vi "Calibrate.vi"(8 "error in (no error)":errorcluster, 11 "Message Queue":refnum<queue>) -> (0 "error out":errorcluster)   [LabVIEW 2020, in "plugin_flodx_ph_probe.lvlib" / "plugin.lvlib"]
doc: "UI which prompts the user to calibrate the device, in two-point and three-point modes."
uses:
  plugin.lvlib
  <userlib>/RxnRover/PluginCore/src/support/Message Queue/Message Cluster.ctl
  <userlib>/RxnRover/PluginCore/src/support/Message Queue/Message Queue.lvlib
panel:
  in  "SHUTDOWN":bool
  in  "Compensation Temperature":sgl=25.0
  in  "Calibrate Button":bool
  in  "Calibration Method":enum32{"TWO-POINT", "THREE-POINT"}(radio)
  in  "Alkaline Buffer pH":sgl=9.8 min=0 format="%#_4g"
  in  "Neutral Buffer pH":sgl=7.01 min=0 format="%#_4g"
  in  "Acidic Buffer pH":sgl=4.1 format="%#_4g"
  in  "Cancel Button":bool
  # "Calibrate Device"
  # "To calibrate your device please input the pH of your buffer solutions used during calibration then choose one of the following options. (If you are only using two out of the three buffer solutions to calibrate leave the unused buffer pH value blank or enter 0)"
  # "Compensation Temperature (C)"
  # "(Calibration Standard 4.10)"
  # "Acidic Buffer(Low)"
  # "(Calibration Standard 7.01)"
  # "Neutral Buffer(Mid)"
  # "(Calibration Standard 9.80)"
  # "Alkaline Buffer(High)"
  # "Calibration Method"
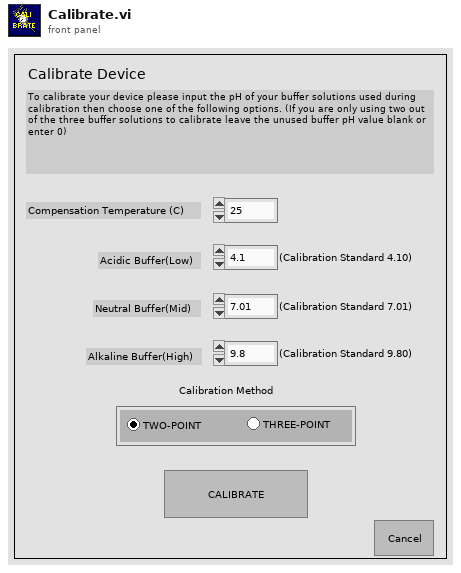
[diagram p1: front panel]
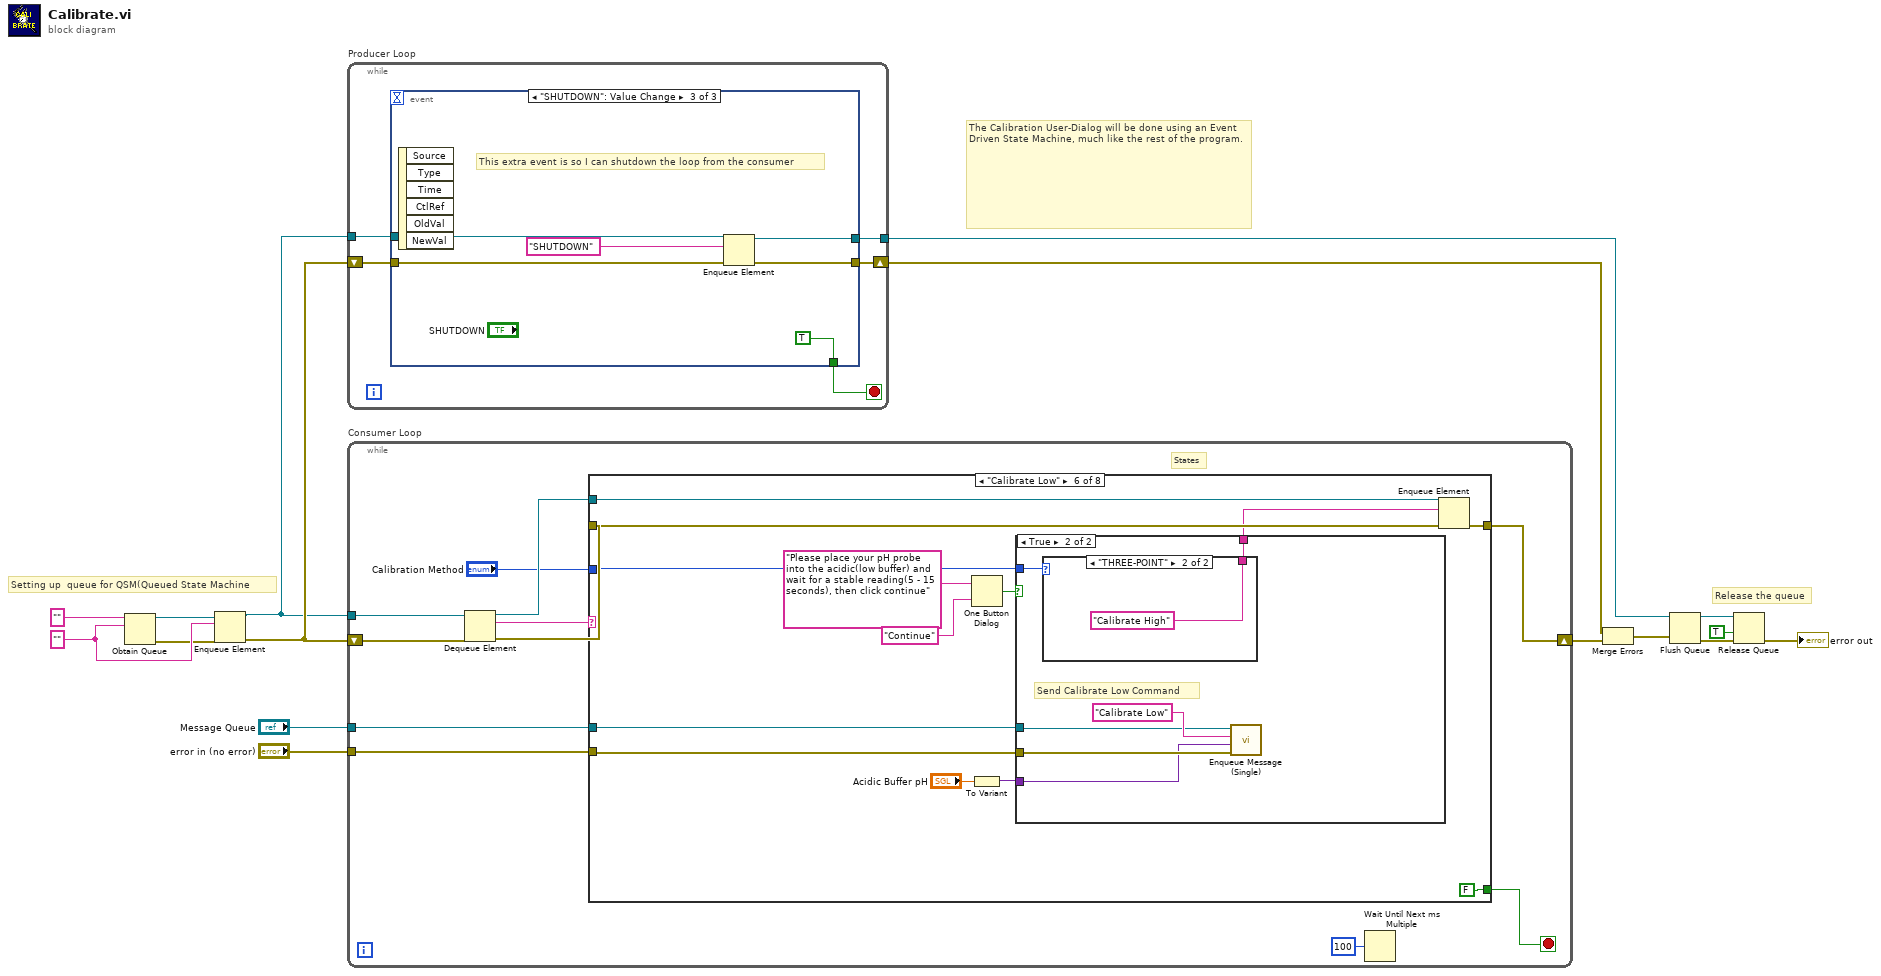
[diagram p0: block diagram]
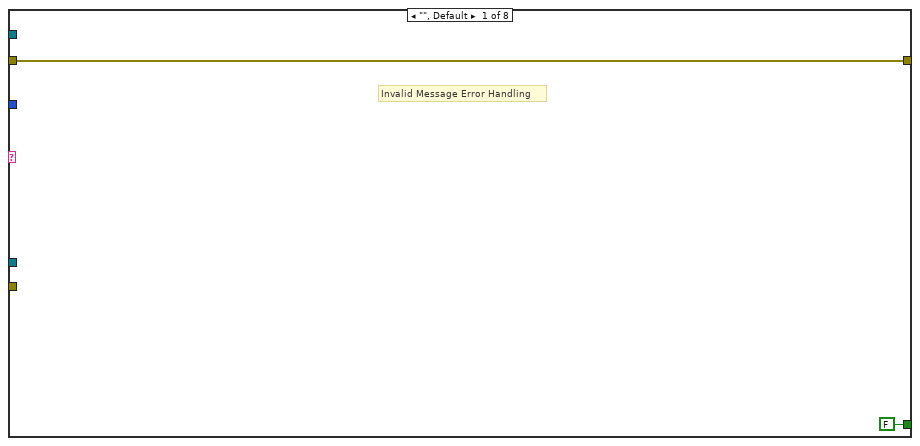
[diagram p2: hidden frame]
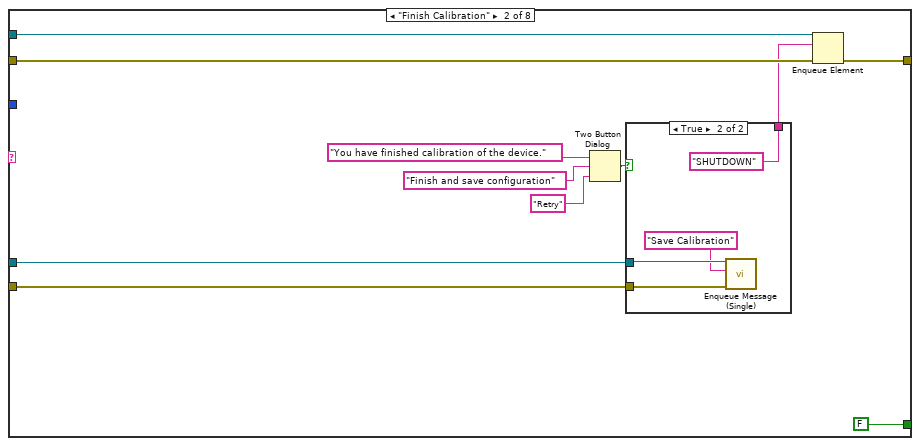
[diagram p3: hidden frame]
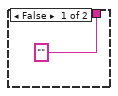
[diagram p4: hidden frame]
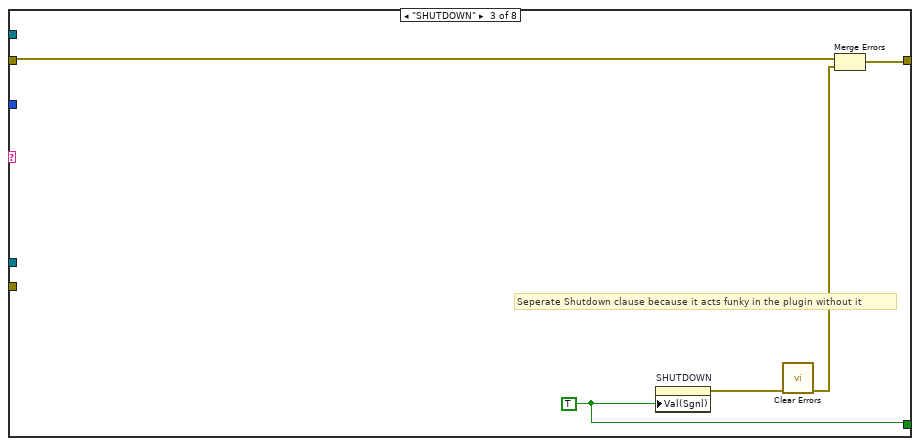
[diagram p5: hidden frame]
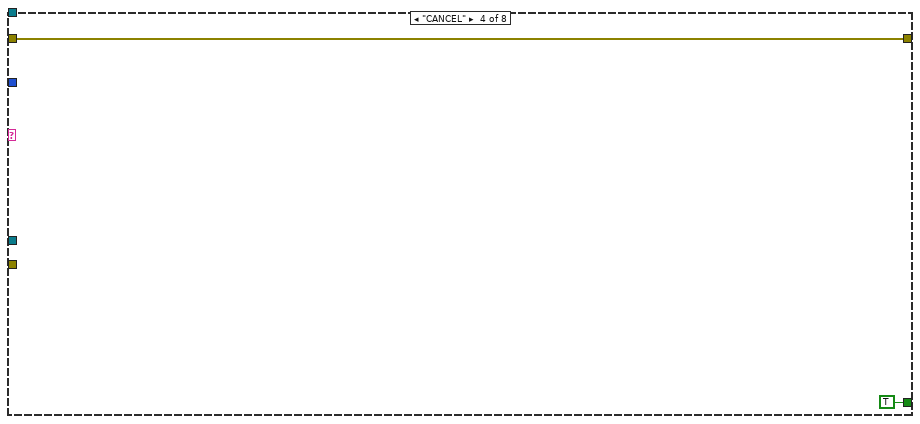
[diagram p6: hidden frame]
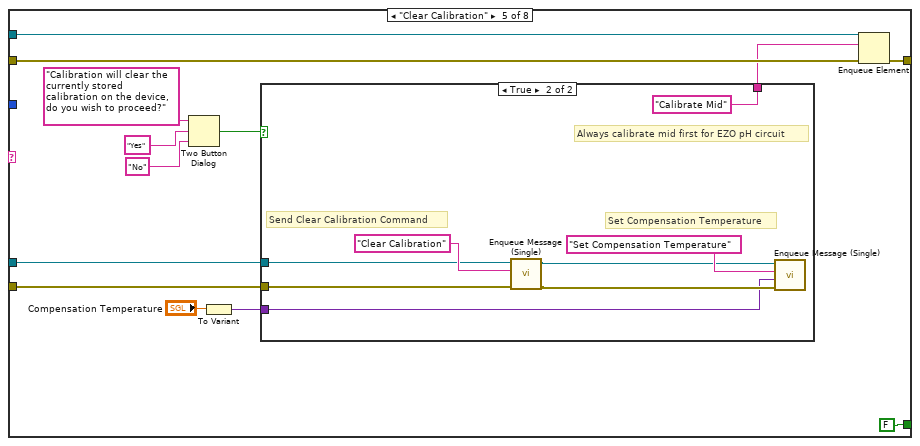
[diagram p7: hidden frame]
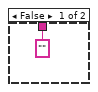
[diagram p8: hidden frame]
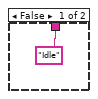
[diagram p9: hidden frame]
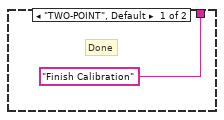
[diagram p10: hidden frame]
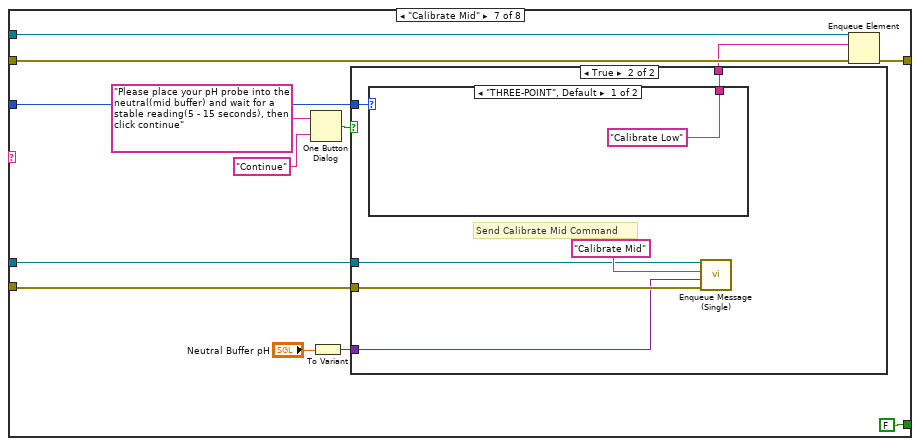
[diagram p11: hidden frame]
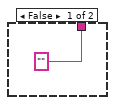
[diagram p12: hidden frame]
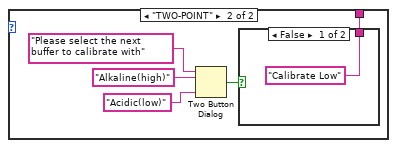
[diagram p13: hidden frame]
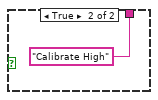
[diagram p14: hidden frame]
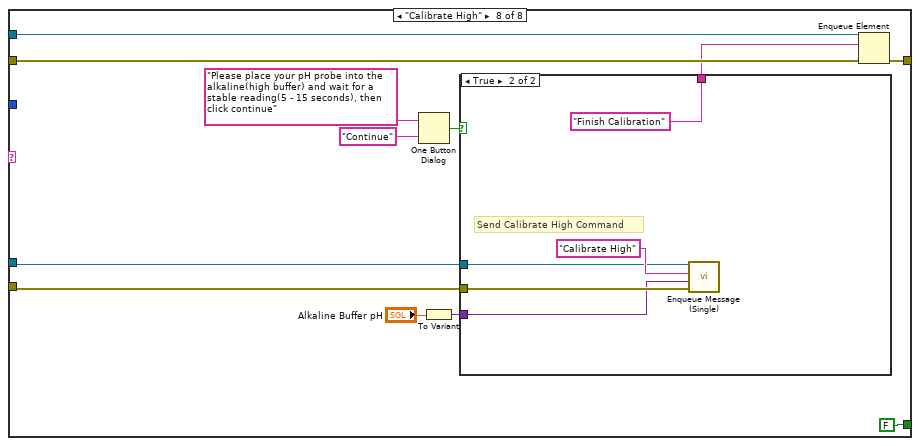
[diagram p15: hidden frame]
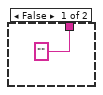
[diagram p16: hidden frame]
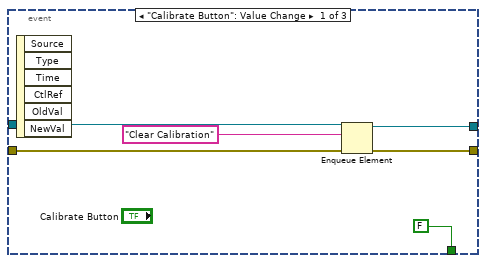
[diagram p17: hidden frame]
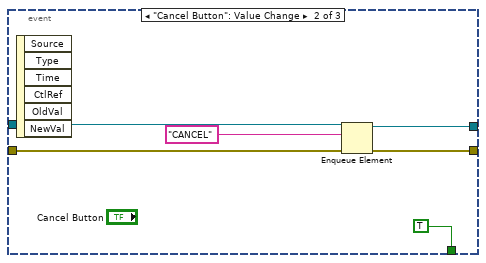
[diagram p18: hidden frame]
diagram:
  w15 = ""
  # "The Calibration User-Dialog will be done using an Event Driven State Machine, much like the rest of the program."
  # "Release the queue"
  # "Setting up  queue for QSM(Queued State Machine"
  n1 = Obtain Queue(name (unnamed)="", element data type=w15) -> (queue out=w14:refnum<queue>, error out=w13:errorcluster)  [unwired: 3 in, 1 out]
  n2 = Enqueue Element(queue=w14, element=w15, error in (no error)=w13) -> (queue out=w1:refnum<queue>, error out=w12:errorcluster)  [unwired: 1 in, 1 out]
  n3 = while "Producer Loop" {
    tunnel: w1 -> [w20]
    shift-right: [w18] -> w8
    shift-left: w12 -> [w21]
    tunnel: [w17] -> w6
    stop <- w19 stop-if-true
    n4 = event shown="[2] \"SHUTDOWN\": Value Change" {
      selector: _ -> [_ _ _]
      dyn-events: _ -> [_ _ _]
      timeout: _ -> [_ _ _]
      tunnel: w21 -> [w27 w33 w39]
      tunnel: w20 -> [w26 w32 w38]
      tunnel: [w25 w31 w37] -> w17
      tunnel: [FALSE TRUE TRUE] -> w19
      tunnel: [w22 w28 w34] -> w18
      event "Calibrate Button": Value Change {
        n5 = event-data() -> ()  [unwired: 1 in, 6 out]
        n6 = Enqueue Element(queue=w26, element="Clear Calibration", error in (no error)=w27) -> (queue out=w25:refnum<queue>, error out=w22:errorcluster)  [unwired: 1 in, 1 out]
      }
      event "Cancel Button": Value Change {
        n7 = event-data() -> ()  [unwired: 1 in, 6 out]
        n8 = Enqueue Element(queue=w32, element="CANCEL", error in (no error)=w33) -> (queue out=w31:refnum<queue>, error out=w28:errorcluster)  [unwired: 1 in, 1 out]
      }
      event "SHUTDOWN": Value Change {
        # "This extra event is so I can shutdown the loop from the consumer"
        n9 = event-data() -> ()  [unwired: 1 in, 6 out]
        n10 = Enqueue Element(queue=w38, element="SHUTDOWN", error in (no error)=w39) -> (queue out=w37:refnum<queue>, error out=w34:errorcluster)  [unwired: 1 in, 1 out]
      }
    }
  }
  n11 = while "Consumer Loop" {
    tunnel: w1 -> [w50]
    tunnel: "Message Queue" -> [w45]
    tunnel: "error in (no error)" -> [w44]
    shift-right: [w41] -> w9
    shift-left: w12 -> [w40]
    stop <- w46 stop-if-true
    # "States"
    n12 = Dequeue Element(queue=w50, error in (no error)=w40) -> (queue out=w48:refnum<queue>, element=w49:string, error out=w47:errorcluster)  [unwired: 1 in, 1 out]
    n13 = case shown="\"Calibrate Low\"" w49 {
      tunnel: w48 -> [_ w58 _ _ w88 w108 w130 w157]
      tunnel: w47 -> [w51 w59 w72 w74 w87 w107 w129 w156]
      tunnel: [FALSE ("T button?") FALSE ("T button?") w69 TRUE ("T button?") FALSE FALSE FALSE FALSE] -> w46
      tunnel: w45 -> [_ w60 _ _ w83 w110 w132 w159]
      tunnel: w44 -> [_ w61 _ _ w84 w109 w131 w158]
      tunnel: "Calibration Method" -> [_ _ _ _ _ w102 w124 _]
      tunnel: [w51 w56 w73 w74 w82 w100 w122 w150] -> w41
      frame "", Default {
        # "Invalid Message Error Handling"
      }
      frame "Finish Calibration" {
        n14 = Two Button Dialog(message="You have finished calibration of the device.", 1:"Retry" ("F button name (\"Cancel\")"), 2:"Finish and save configuration" ("T button name (\"OK\")")) -> (T button?=w55:bool)
        n15 = case shown="True" w55 {
          tunnel: w61 -> [_ w68]
          tunnel: w60 -> [_ w67]
          tunnel: ["" ("element") "SHUTDOWN" ("element")] -> w57
          frame False {
          }
          frame True {
            n16 = call <userlib>:"Enqueue Message (Single).vi"("error in (no error)"=w68, "Message"="Save Calibration", "Message Queue"=w67) -> ()  [unwired: 7 in, 2 out]
          }
        }
        n17 = Enqueue Element(queue=w58, element=w57, error in (no error)=w59) -> (error out=w56:errorcluster)  [unwired: 1 in, 2 out]
      }
      frame "SHUTDOWN" {
        w69 = TRUE
        # "Seperate Shutdown clause because it acts funky in the plugin without it"
        n18 = property on="SHUTDOWN" class="Bool (strict)"("Val(Sgnl)"=w69) -> (error out=w70:errorcluster)  [unwired: 2 in, 1 out]
        n19 = call <vilib>:"Clear Errors.vi"("error in (no error)"=w70) -> ("error out"=w71:errorcluster)  [unwired: 5 in, 1 out]
        n20 = Merge Errors(w72, w71) -> (w73:errorcluster)
      }
      frame "CANCEL" {
      }
      frame "Clear Calibration" {
        n21 = Two Button Dialog(message="Calibration will clear the currently stored calibration on the device, do you wish to proceed?", 1:"No" ("F button name (\"Cancel\")"), 2:"Yes" ("T button name (\"OK\")")) -> (T button?=w79:bool)
        n22 = To Variant(anything="Compensation Temperature") -> (Variant=w80:variant)
        n23 = case shown="True" w79 {
          tunnel: ["" ("element") "Calibrate Mid" ("element")] -> w86
          tunnel: w84 -> [_ w94]
          tunnel: w83 -> [_ w91]
          tunnel: w80 -> [_ w90]
          frame False {
          }
          frame True {
            # "Send Clear Calibration Command"
            # "Always calibrate mid first for EZO pH circuit"
            # "Set Compensation Temperature"
            n24 = call <userlib>:"Enqueue Message (Single).vi"("error in (no error)"=w94, "Message"="Clear Calibration", "Message Queue"=w91) -> ("error out"=w93:errorcluster, "dup Message Queue"=w92:refnum<queue>)  [unwired: 7 in]
            n25 = call <userlib>:"Enqueue Message (Single).vi"("error in (no error)"=w93, "Message Data"=w90, "Message"="Set Compensation Temperature", "Message Queue"=w92) -> ()  [unwired: 6 in, 2 out]
          }
        }
        n26 = Enqueue Element(queue=w88, element=w86, error in (no error)=w87) -> (error out=w82:errorcluster)  [unwired: 1 in, 2 out]
      }
      frame "Calibrate Low" {
        n27 = One Button Dialog(message="Please place your pH probe into the acidic(low buffer) and wait for a stable reading(5 - 15 seconds), then click continue", button name ("OK")="Continue") -> (true=w103:bool)
        n28 = To Variant(anything="Acidic Buffer pH") -> (Variant=w98:variant)
        n29 = case shown="True" w103 {
          tunnel: w110 -> [_ w116]
          tunnel: w109 -> [_ w115]
          tunnel: ["Idle" ("element") w114] -> w106
          tunnel: w102 -> [_ w113]
          tunnel: w98 -> [_ w112]
          frame False {
          }
          frame True {
            # "Send Calibrate Low Command"
            n30 = case shown="\"THREE-POINT\"" w113 {
              tunnel: ["Finish Calibration" ("element") "Calibrate High" ("element")] -> w114
              frame "TWO-POINT", Default {
                # "Done"
              }
              frame "THREE-POINT" {
              }
            }
            n31 = call <userlib>:"Enqueue Message (Single).vi"("error in (no error)"=w115, "Message Data"=w112, "Message"="Calibrate Low", "Message Queue"=w116) -> ()  [unwired: 6 in, 2 out]
          }
        }
        n32 = Enqueue Element(queue=w108, element=w106, error in (no error)=w107) -> (error out=w100:errorcluster)  [unwired: 1 in, 2 out]
      }
      frame "Calibrate Mid" {
        n33 = One Button Dialog(message="Please place your pH probe into the neutral(mid buffer) and wait for a stable reading(5 - 15 seconds), then click continue", button name ("OK")="Continue") -> (true=w125:bool)
        n34 = To Variant(anything="Neutral Buffer pH") -> (Variant=w120:variant)
        n35 = case shown="True" w125 {
          tunnel: w132 -> [_ w138]
          tunnel: w131 -> [_ w137]
          tunnel: ["" ("element") w136] -> w128
          tunnel: w124 -> [_ w135]
          tunnel: w120 -> [_ w134]
          frame False {
          }
          frame True {
            # "Send Calibrate Mid Command"
            n36 = case shown="\"THREE-POINT\", Default" w135 {
              tunnel: ["Calibrate Low" ("element") w141] -> w136
              frame "THREE-POINT", Default {
              }
              frame "TWO-POINT" {
                n37 = Two Button Dialog(message="Please select the next buffer to calibrate with", 1:"Acidic(low)" ("F button name (\"Cancel\")"), 2:"Alkaline(high)" ("T button name (\"OK\")")) -> (T button?=w142:bool)
                n38 = case shown="False" w142 {
                  tunnel: ["Calibrate Low" ("element") "Calibrate High" ("element")] -> w141
                  frame False {
                  }
                  frame True {
                  }
                }
              }
            }
            n39 = call <userlib>:"Enqueue Message (Single).vi"("error in (no error)"=w137, "Message Data"=w134, "Message"="Calibrate Mid", "Message Queue"=w138) -> ()  [unwired: 6 in, 2 out]
          }
        }
        n40 = Enqueue Element(queue=w130, element=w128, error in (no error)=w129) -> (error out=w122:errorcluster)  [unwired: 1 in, 2 out]
      }
      frame "Calibrate High" {
        n41 = One Button Dialog(message="Please place your pH probe into the alkaline(high buffer) and wait for a stable reading(5 - 15 seconds), then click continue", button name ("OK")="Continue") -> (true=w152:bool)
        n42 = To Variant(anything="Alkaline Buffer pH") -> (Variant=w148:variant)
        n43 = case shown="True" w152 {
          tunnel: w159 -> [_ w164]
          tunnel: w158 -> [_ w163]
          tunnel: ["" ("element") "Finish Calibration" ("element")] -> w155
          tunnel: w148 -> [_ w161]
          frame False {
          }
          frame True {
            # "Send Calibrate High Command"
            n44 = call <userlib>:"Enqueue Message (Single).vi"("error in (no error)"=w163, "Message Data"=w161, "Message"="Calibrate High", "Message Queue"=w164) -> ()  [unwired: 6 in, 2 out]
          }
        }
        n45 = Enqueue Element(queue=w157, element=w155, error in (no error)=w156) -> (error out=w150:errorcluster)  [unwired: 1 in, 2 out]
      }
    }
    n46 = Wait Until Next ms Multiple(millisecond multiple=u32 100) -> ()  [unwired: 1 out]
  }
  n47 = Merge Errors(w8, w9) -> (w4:errorcluster)
  n48 = Flush Queue(queue=w6, error in (no error)=w4) -> (queue out=w5:refnum<queue>, error out=w3:errorcluster)  [unwired: 1 out]
  n49 = Release Queue(queue=w5, force destroy? (F)=TRUE, error in (no error)=w3) -> (error out=→"error out":errorcluster)  [unwired: 2 out]
